vi "Read Process Variable.vi"(8 "error in (no error)":errorcluster, 10 "Process Variable":u32=1 min=1 step=1, 11 "F4T in":refnum<class "F4T.lvclass">) -> (0 "error out":errorcluster, 2 "Value":dbl, 3 "F4T out":refnum<class "F4T.lvclass">)   [LabVIEW 2018, in "F4T.lvlib" / "F4T.lvclass"]
doc: "This Override is used to read a Process Variable value."
uses:
  F4T.lvclass
  Custom Controls/Command Data.ctl
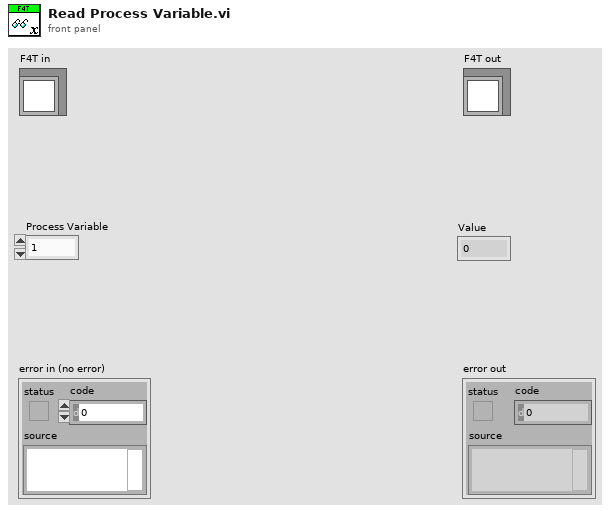
[diagram p1: front panel]
types:
  T1 = typedef "F4T.lvlib/F4T.lvclass/Command Data.ctl" = cluster{"ParameterID":u32, "InstanceId":u32, "Value":string}
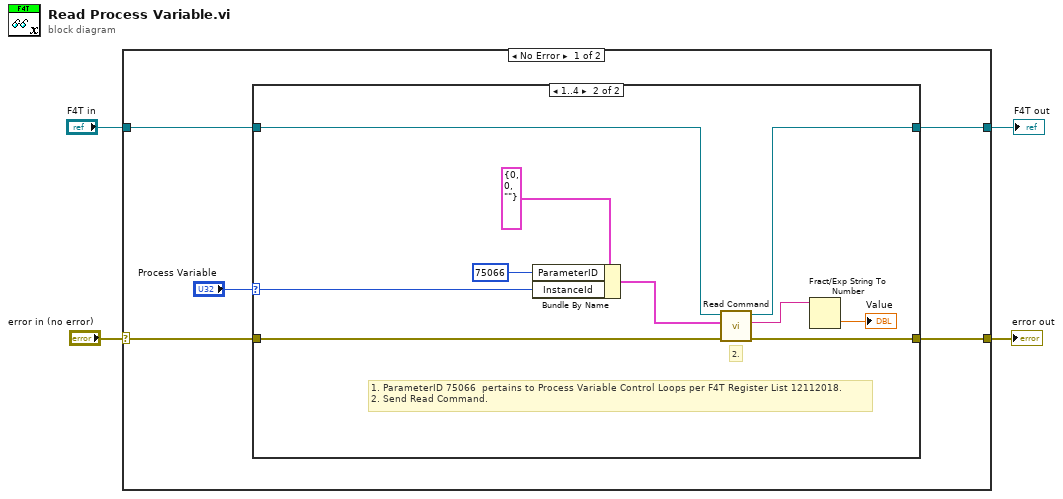
[diagram p0: block diagram]
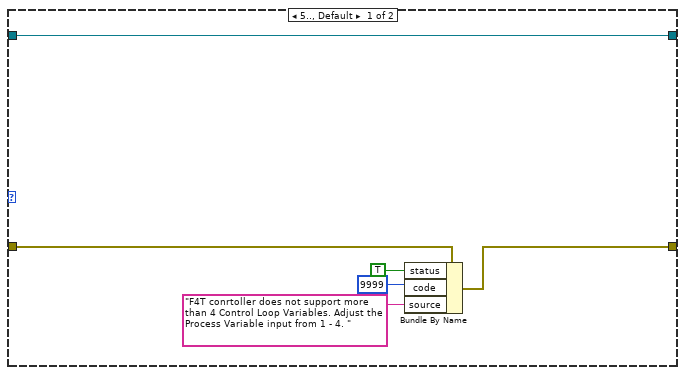
[diagram p2: hidden frame]
diagram:
  n1 = case shown="No Error" "error in (no error)" {
    selector: "error in (no error)" -> [w9 w27]
    tunnel: [w8 w27] -> w3
    tunnel: [w7 w26] -> w2
    tunnel: "F4T in" -> [w6 w26]
    frame No Error {
      n2 = case shown="1..4" "Process Variable" {
        selector: "Process Variable" -> [_ w18]
        tunnel: w9 -> [w14 w25]
        tunnel: [w13 w24] -> w8
        tunnel: [w15 w23] -> w7
        tunnel: w6 -> [w15 w20]
        frame 5.., Default {
          n3 = Bundle By Name(cluster=w14, "status"=TRUE, "code"=9999, "source"="F4T conrtoller does not support more than 4 Control Loop Variables. Adjust the Process Variable input from 1 - 4. ") -> (w13:errorcluster)
        }
        frame 1..4 {
          # "1. ParameterID 75066  pertains to Process Variable Control Loops per F4T Register List 12112018.\n2. Send Read Command."
          # "2."
          n4 = Bundle By Name(cluster=T1 {"ParameterID"=0, "InstanceId"=0, "Value"=""} ("Command Data"), "ParameterID"=u32 75066, "InstanceId"=w18) -> (w16:T1)
          n5 = call "Read Command.vi"("error in (no error)"=w25, "Command Data"=w16, "F4T in"=w20) -> ("error out"=w24:errorcluster, "Response"=w22:string, "F4T out"=w23:refnum<class "F4T.lvclass">)  [unwired: 6 in]
          n6 = Fract/Exp String To Number(string=w22) -> (number=→"Value":dbl)  [unwired: 3 in, 1 out]
        }
      }
    }
    frame Error {
    }
  }
  "error out" <- w3
  "F4T out" <- w2
